vi "UniqueArrayNumU32.vi"(8 "Input Array":u32[](array[numeric])) -> (2 "Output Array":u32[](array[numeric]))   [LabVIEW 2017, in "AppPlugins.lvlib" / "LSEPlugin.lvclass"]
doc: "This VI takes an Input of an Array and removes all duplicate entries, and returns an array with every element unique."
uses:
  LSEPlugin.lvclass
panel:
  # "Christian Altenbach, 2009 see discussion:\nhttp://decibel.ni.com/content/docs/DOC-4882"
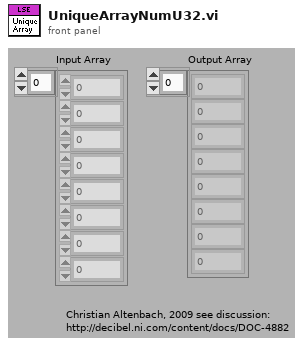
[diagram p1: front panel]
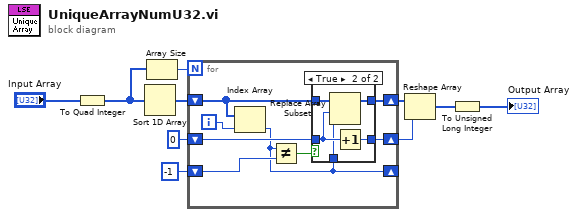
[diagram p0: block diagram]
diagram:
  n1 = To Quad Integer(1:"Input Array") -> (0:w2:i64[])
  n2 = Sort 1D Array(array=w2) -> (sorted array=w10:i64[])
  n3 = Array Size(array=w2) -> (size(s)=w6:i32)
  n4 = for {
    N: w6 -> [_]
    shift-right: [w14] -> w8
    shift-left: w10 -> [w13]
    shift-right: [w11] -> _
    shift-left: i64 -1 ("Numeric 3") -> [w18]
    shift-right: [w15] -> w7
    shift-left: 0 -> [w16]
    i -> [w12]
    n5 = Index Array(array=w13, index=w12) -> (element=w11:i64)
    n6 = Not Equal?(x=w11, y=w18) -> (x != y?=w17:bool)
    n7 = case shown="True" w17 {
      tunnel: w16 -> [w20 w24]
      tunnel: [w20 w25] -> w15
      tunnel: w11 -> [_ w23]
      tunnel: w13 -> [w19 w22]
      tunnel: [w19 w21] -> w14
      frame False {
      }
      frame True {
        n8 = Replace Array Subset(array=w22, new element=w23, index=w24) -> (w21:i64[])
        n9 = Increment(x=w24) -> (x+1=w25:i32)
      }
    }
  }
  n10 = Reshape Array(w8, w7) -> (w4:i64[])
  n11 = To Unsigned Long Integer(number=w4) -> (unsigned 32bit integer=→"Output Array":u32[])
